vi "Get Selected Sites.vi"(8 "error in (no error)":errorcluster, 11 "Session in":refnum<class "Plugin Session.lvclass">) -> (0 "error out":errorcluster, 2 "Selected Sites":i32[](array[numeric]), 3 "Session out":refnum<class "Plugin Session.lvclass">)   [LabVIEW 2021, in "InstrumentStudio Plugin SDK.lvlib" / "Plugin Session.lvclass"]
doc: "Call this VI to read the list of selected sites being displayed within InstrumentStudio. If the active pin \nmap does not exist or is invalid, an empty list will be returned."
uses:
  Plugin Session.lvclass
  Plugin Session.lvclass/Plugin Session.ctl
  Read Session Id.vi
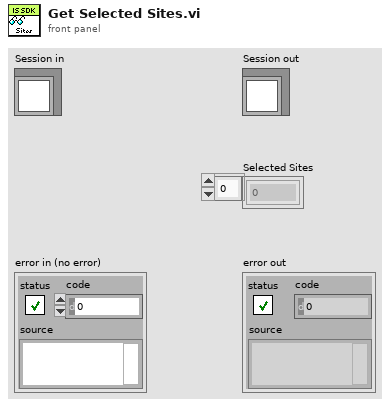
[diagram p1: front panel]
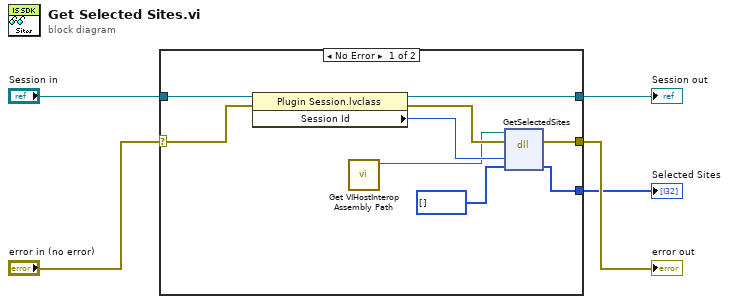
[diagram p0: block diagram]
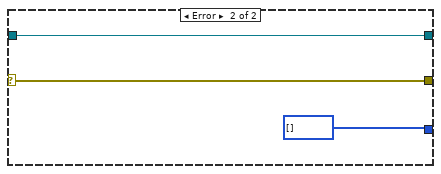
[diagram p2: hidden frame]
diagram:
  n1 = case shown="No Error" "error in (no error)" {
    selector: "error in (no error)" -> [w12 w16]
    tunnel: "Session in" -> [w14 w17]
    tunnel: [w13 w17] -> w5
    tunnel: [w9 w16] -> w2
    tunnel: [w6 i32[] [] ("sites")] -> w1
    frame No Error {
      n2 = property class="Plugin Session.lvclass"(reference=w14, error in=w12) -> (reference out=w13:refnum<class "Plugin Session.lvclass">, error out=w11:errorcluster, "Session Id"=w10:u64)
      n3 = call "Get VIHostInterop Assembly Path.vi"() -> ("VIHost.Interop Assembly"=w7:path)  [unwired: 11 in]
      n4 = dll-call lib="C:/Dev/ASW/Source/InstrumentStudio/IFDistribution/VIHostPanel/objects/export/targets/win64U/x64/msvc-14.0/debug/NationalInstruments.VIHost.Interop.dll" fn="GetSelectedSites"(path in=w7, error in=w11, "sessionId"=w10, "sites"=i32[] []) -> (error out=w9:errorcluster, "sites"=w6:i32[])  [unwired: 3 in, 1 out]
    }
    frame Error {
    }
  }
  "error out" <- w2
  "Session out" <- w5
  "Selected Sites" <- w1
